vi "FPGA.vi"() -> ()   [LabVIEW 2019]
uses:
  <vilib>/eio/EIONode/EIONode.xnode
  <vilib>/rvi/eio/common/nirviEmuTemplateMethod_errors.vi
panel:
  out "AudioIn/Right":i16
  out "AudioIn/Left":i16
  out "ConnectorC/DIO7:0":u8
  in  "ConnectorC/AO1":i16
  out "Button0":bool
  out "ConnectorC/AI1":i16
  out "ConnectorC/AI0":i16
  in  "ConnectorC/DIO7":bool
  in  "AudioOut/Right":i16
  in  "AudioOut/Left":i16
  out "AccelerationX":i16
  out "AccelerationY":i16
  out "AccelerationZ":i16
  out "Scan Clock":bool
  in  "LED3":bool
  in  "LED2":bool
  in  "LED1":bool
  in  "LED0":bool
  in  "ConnectorC/DIO0":bool
  in  "ConnectorC/DIO3":bool
  in  "ConnectorC/AO0":i16
  in  "ConnectorC/DIO2":bool
  in  "ConnectorC/DIO4":bool
  in  "ConnectorC/DIO5":bool
  in  "ConnectorC/DIO6":bool
  in  "System Reset":bool
  # "on board"
  # "Audio"
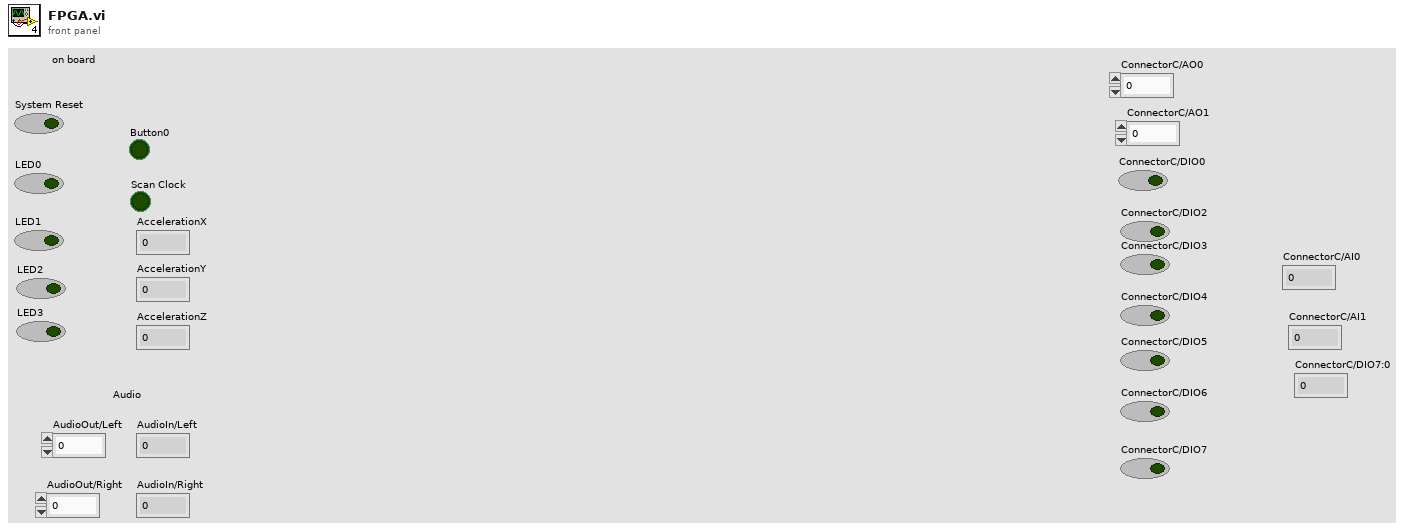
[diagram p1: front panel]
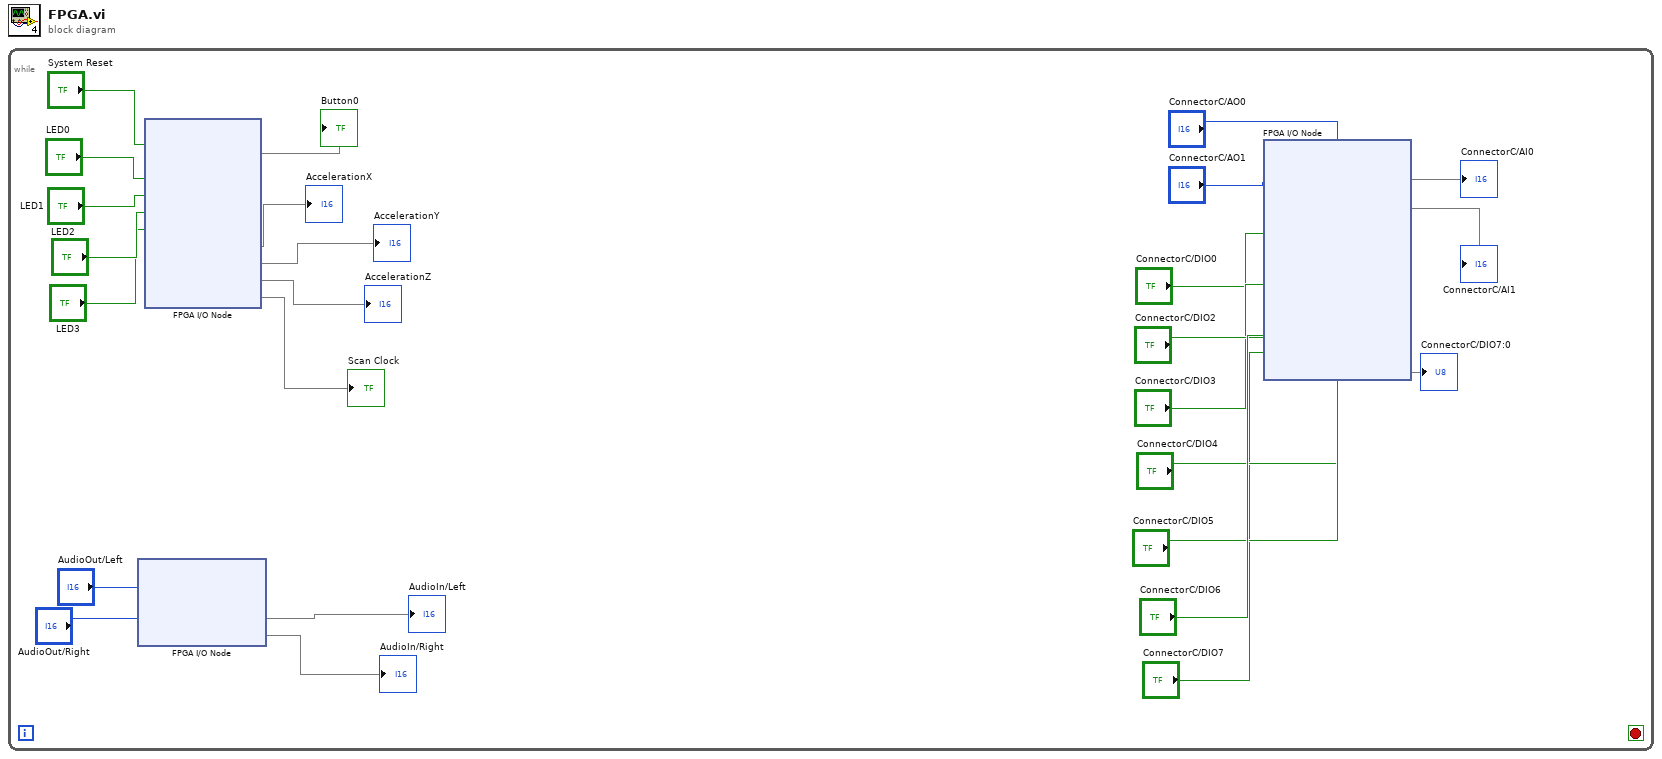
[diagram p0: block diagram]
diagram:
  n1 = while {
    stop <- _ stop-if-true
    n2 = xnode "FPGA I/O Node"("AudioOut/Left"="AudioOut/Left", "AudioOut/Right"="AudioOut/Right") -> ("AudioIn/Left"=→"AudioIn/Left", "AudioIn/Right"=→"AudioIn/Right")  [unwired: 4 in, 4 out]
    n3 = xnode "FPGA I/O Node"("System Reset"="System Reset", "LED0"="LED0", "LED1"="LED1", "LED2"="LED2", "LED3"="LED3") -> ("Button0"=→"Button0", "AccelerationX"=→"AccelerationX", "AccelerationY"=→"AccelerationY", "AccelerationZ"=→"AccelerationZ", "Scan Clock"=→"Scan Clock")  [unwired: 10 in, 10 out]
    n4 = xnode "FPGA I/O Node"("ConnectorC/AO0"="ConnectorC/AO0", "ConnectorC/AO1"="ConnectorC/AO1", "ConnectorC/DIO0"="ConnectorC/DIO0", "ConnectorC/DIO2"="ConnectorC/DIO2", "ConnectorC/DIO3"="ConnectorC/DIO3", "ConnectorC/DIO4"="ConnectorC/DIO4", "ConnectorC/DIO5"="ConnectorC/DIO5", "ConnectorC/DIO6"="ConnectorC/DIO6", "ConnectorC/DIO7"="ConnectorC/DIO7") -> ("ConnectorC/AI0"=→"ConnectorC/AI0", "ConnectorC/AI1"=→"ConnectorC/AI1", "ConnectorC/DIO7:0"=→"ConnectorC/DIO7:0")  [unwired: 14 in, 13 out]
  }
